vi "Main-loop-backup.vi"() -> ()   [LabVIEW 2016]
uses:
  Sched_state.ctl
  Plant_info.ctl
  <vilib>/Platform/TimedLoop/XDataNode/timing_clust.ctl
  <vilib>/Platform/TimedLoop/XDataNode/nitl_modes.ctl
  <vilib>/Platform/TimedLoop/XDataNode/wakeup.ctl
  <vilib>/Platform/TimedLoop/XDataNode/XDataNode.xnode
  <vilib>/Platform/TimedLoop/XDataNode/XDNodeRunTimeDep.lvlib
panel:
  out "error out":errorcluster
  out "loop time\n(only for diagnostics) - should be exactly 10, always":u32
  out "Plant 2 region":dbl(graph)
  out "Plant 1 region":dbl(graph)
  out "Plant 2":cluster{"Input":dbl, "Data":dbl, "Data":dbl}(graph)
  out "Plant 1":cluster{"Input":dbl, "Data":dbl, "Data":dbl}(graph)
  in  "error in (no error)":errorcluster
  in  "stop main":bool
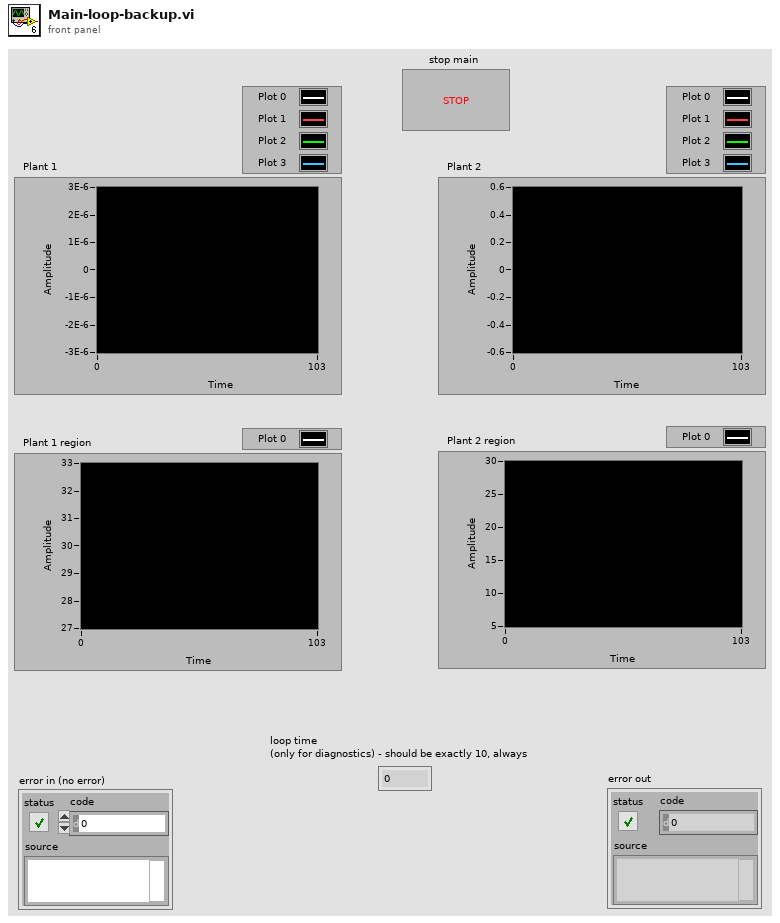
[diagram p1: front panel]
types:
  T1 = typedef "Sched_state.ctl" = cluster{"Plant 1":T2, "Plant 2":T2}
  T2 = typedef "Plant_info.ctl" = cluster{"Clk":dbl, "Region":dbl, "Input":dbl}
  T3 = typedef "Plant-data.ctl" = cluster{"Plant X1 ":dbl[], "Plant X2":dbl[], "Plant K*x_hat":dbl[], "Region":i32[]}
  T4 = typedef "XDNodeRunTimeDep.lvlib/timing_clust.ctl" = cluster{"Expected End [f-1]":u64, "Actual End [f-1]":u64, "Finished Late? [f-1]":bool, "Expected End [i-1]":u64, "Actual End [i-1]":u64, "Finished Late? [i-1]":bool, "Expected Start [i]":u64, "Actual Start [i]":u64, "Expected Start [f]":u64, "Actual Start [f]":u64, "Source Name":string, "Structure Name":string, "Period":i64, "Deadline":i64, "Offset":i64, "Start":i64, "Priority":i32, "Timeout":i32, "Mode":T5, "Wakeup Reason":T6, "Error":errorcluster, "Source Type":string, "Secondary Source Type":string, "Global End Time":u64, "Global Start Time":u64, "Frame Duration":u64, "Iteration Duration":u64, "Assigned CPU":i32, "I/O Scan Engine Mode":u32}
  T5 = typedef "XDNodeRunTimeDep.lvlib/nitl_modes.ctl" = enum32{"No Change", "Process missed periods, maintain original phase", "Discard missed periods, maintain original phase", "Process missed periods, ignore original phase", "Discard missed periods, ignore original phase"}
  T6 = typedef "XDNodeRunTimeDep.lvlib/wakeup.ctl" = enum32{"Normal", "Aborted", "Asynchronous wakeup", "Timing source error", "Timed loop error", "Timeout"}
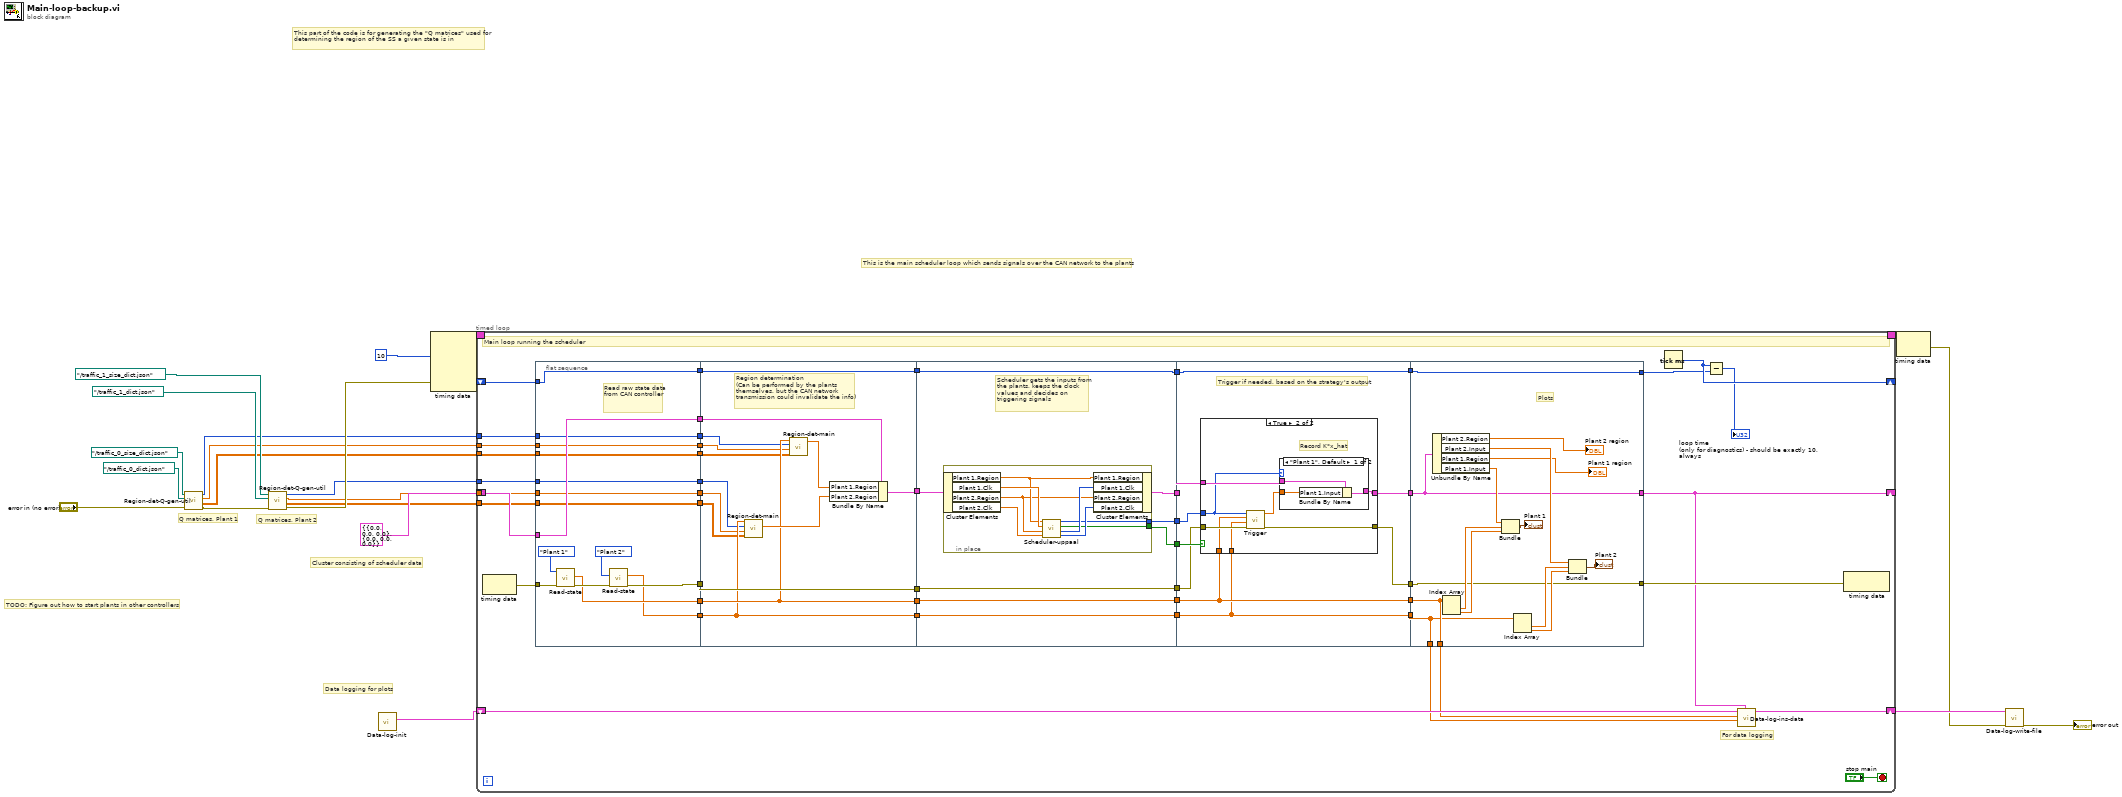
[diagram p0: block diagram]
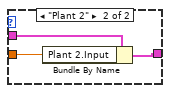
[diagram p3: hidden frame]
diagram:
  # "Data logging for plots"
  # "Q matrices, Plant 2"
  # "Q matrices, Plant 1"
  # "Cluster consisting of scheduler data"
  # "This part of the code is for generating the \"Q matrices\" used for determining the region of the SS a given state is in"
  # "TODO: Figure out how to start plants in other controllers"
  # "This is the main scheduler loop which sends signals over the CAN network to the plants"
  n1 = call "Region-det-Q-gen-util.vi"("error in"="error in (no error)", "Actual Q matrix JSON - rel path"=path "../traffic_0_dict.json", "Q matrix info JSON - rel path"=path "../traffic_0_size_dict.json") -> ("error out"=w13:errorcluster, "Q Matrices"=w6:dbl[][][][], "Index array"=w7:dbl[], "Regions"=w8:i32[])  [unwired: 5 in]
  n2 = call "Region-det-Q-gen-util.vi"("error in"=w13, "Actual Q matrix JSON - rel path"=path "../traffic_1_dict.json", "Q matrix info JSON - rel path"=path "../traffic_1_size_dict.json") -> ("error out"=w12:errorcluster, "Q Matrices"=w9:dbl[][][][], "Index array"=w5:dbl[], "Regions"=w10:i32[])  [unwired: 5 in]
  n3 = call "Data-log-init.vi"() -> ("Data cluster"=w4:cluster{"Plant 2":T3, "Plant 1":T3})  [unwired: 10 in, 1 out]
  n4 = node-c288(i64 10 ("Period"), w12) -> (w21:T4)  [unwired: 3 in]
  n5 = timed-loop {
    timing: w21 -> [_]
    timing-out: [_] -> w20
    shift-right: [w22] -> _
    shift-left: T1 {"Plant 1"={"Clk"=0.0, "Region"=0.0, "Input"=0.0}, "Plant 2"={"Clk"=0.0, "Region"=0.0, "Input"=0.0}} ("Scheduler State") -> [w65]
    tunnel: w10 -> [w47]
    tunnel: w5 -> [w44]
    tunnel: w9 -> [w42]
    tunnel: w8 -> [w40]
    tunnel: w7 -> [w39]
    tunnel: w6 -> [w36]
    shift-right: [w34] -> _
    shift-left: _ -> [w32]
    shift-right: [w25] -> w3
    shift-left: w4 -> [w26]
    stop <- "stop main" stop-if-true
    # "For data logging"
    # "Main loop running the scheduler"
    n6 = node-c288() -> (w68:errorcluster)  [unwired: 1 in]
    n7 = flat-sequence {
      tunnel: w68 -> [w81]
      tunnel: w65 -> [w78]
      tunnel: [w78] -> w56
      tunnel: [w79] -> w52
      tunnel: [w77] -> w49
      tunnel: [w76] -> w48
      tunnel: w47 -> [w75]
      tunnel: [w75] -> w46
      tunnel: [w74] -> w45
      tunnel: w44 -> [w74]
      tunnel: [w73] -> w43
      tunnel: w42 -> [w73]
      tunnel: [w72] -> w41
      tunnel: w40 -> [w72]
      tunnel: w39 -> [w71]
      tunnel: [w71] -> w38
      tunnel: w36 -> [w70]
      tunnel: [w70] -> w37
      tunnel: w32 -> [w69]
      tunnel: [w69] -> w31
      tunnel: [w92] -> w62
      tunnel: [w91] -> w59
      tunnel: w56 -> [w97]
      tunnel: [w94] -> w55
      tunnel: [w93] -> w53
      tunnel: w52 -> [w93]
      tunnel: w49 -> [w92]
      tunnel: w48 -> [w91]
      tunnel: w46 -> [w90]
      tunnel: w45 -> [w89]
      tunnel: w43 -> [w88]
      tunnel: w41 -> [w87]
      tunnel: w38 -> [w85]
      tunnel: w37 -> [w86]
      tunnel: w31 -> [w84]
      tunnel: [w84] -> w30
      tunnel: [w105] -> w64
      tunnel: [w99] -> w63
      tunnel: w62 -> [w104]
      tunnel: [w104] -> w61
      tunnel: [w103] -> w60
      tunnel: w59 -> [w103]
      tunnel: [w102] -> w57
      tunnel: w55 -> [w101]
      tunnel: [w100] -> w54
      tunnel: w53 -> [w100]
      tunnel: w30 -> [w98]
      tunnel: [w98] -> w28
      tunnel: [w119] -> w67
      tunnel: w64 -> [w115]
      tunnel: w63 -> [w120]
      tunnel: w61 -> [w117]
      tunnel: w60 -> [w116]
      tunnel: [w121] -> w58
      tunnel: w57 -> [w122]
      tunnel: w54 -> [w118]
      tunnel: [w116] -> w51
      tunnel: [w117] -> w50
      tunnel: [w114] -> w29
      tunnel: w28 -> [w114]
      tunnel: w67 -> [w143]
      tunnel: [w142] -> w22
      tunnel: w58 -> [w142]
      tunnel: w51 -> [w139]
      tunnel: w50 -> [w140]
      tunnel: [w143] -> w35
      tunnel: [w141] -> w33
      tunnel: w29 -> [w141]
      tunnel: [w140] -> w24
      tunnel: [w139] -> w23
      frame #0 {
        # "Read raw state data from CAN controller"
        n8 = call "Read-state.vi"("error in (no error)"=w81, "Plant"=enum16{"Plant 1", "Plant 2"}."Plant 1") -> ("error out"=w80:errorcluster, "state"=w77:dbl[])  [unwired: 8 in]
        n9 = call "Read-state.vi"("error in (no error)"=w80, "Plant"=enum16{"Plant 1", "Plant 2"}."Plant 2") -> ("error out"=w79:errorcluster, "state"=w76:dbl[])  [unwired: 8 in]
      }
      frame #1 {
        # "Region determination \n(Can be performed by the plants\nthemselves, but the CAN network \ntransmission could invalidate the info)"
        n10 = call "Region-det-main.vi"("Q Matrices"=w88, "Index Array"=w89, "Regions"=w90, "State"=w91) -> ("Region"=w95:dbl)  [unwired: 7 in]
        n11 = call "Region-det-main.vi"("Q Matrices"=w86, "Index Array"=w85, "Regions"=w87, "State"=w92) -> ("Region"=w96:dbl)  [unwired: 7 in]
        n12 = Bundle By Name(cluster=w97, "Plant 1.Region"=w96, "Plant 2.Region"=w95) -> (w94:T1)
      }
      frame #2 {
        # "Scheduler gets the inputs from the plants, keeps the clock values and decides on triggering signals"
        n13 = in-place {
          in-place-border: [w111] -> w105
          in-place-border: [w110] -> w99
          n14 = in-place-cluster #1(w101) -> ("Plant 1.Region"=w107:dbl, "Plant 1.Clk"=w109:dbl, "Plant 2.Region"=w106:dbl, "Plant 2.Clk"=w108:dbl)
          n15 = call "Scheduler-uppaal.vi"("Clock, plant 2"=w108, "Region, plant 2"=w106, "Clock, plant 1"=w109, "Region, plant 1"=w107) -> ("Clock 2"=w112:i32, "Clock 1"=w113:i32, "Trigger?"=w110:bool, "Plant to trigg"=w111:enum16{"Plant 1", "Plant 2"})  [unwired: 4 in]
          n16 = in-place-cluster #1("Plant 1.Region"=w107, "Plant 1.Clk"=w113, "Plant 2.Region"=w106, "Plant 2.Clk"=w112) -> (w102:T1)
        }
      }
      frame #3 {
        # "Trigger if needed, based on the strategy's output"
        n17 = case shown="True" w120 {
          tunnel: w122 -> [w124 w129]
          tunnel: [w124 w130] -> w121
          tunnel: w117 -> [_ w126]
          tunnel: w118 -> [w123 w132]
          tunnel: [w123 w131] -> w119
          tunnel: w115 -> [_ w128]
          tunnel: w116 -> [_ w125]
          frame False {
          }
          frame True {
            # "Record K*x_hat"
            n18 = call "Trigger.vi"("error in (no error)"=w132, "State, Plant 2"=w125, "State, Plant 1"=w126, "Plant to trigg"=w128) -> ("error out"=w131:errorcluster, "Kx"=w127:dbl)  [unwired: 6 in]
            n19 = case shown="\"Plant 1\", Default" w128 {
              tunnel: [w133 w138] -> w130
              tunnel: w129 -> [w135 w137]
              tunnel: w127 -> [w134 w136]
              frame "Plant 1", Default {
                n20 = Bundle By Name(cluster=w135, "Plant 1.Input"=w134) -> (w133:T1)
              }
              frame "Plant 2" {
                n21 = Bundle By Name(cluster=w137, "Plant 2.Input"=w136) -> (w138:T1)
              }
            }
          }
        }
      }
      frame #4 {
        # "Plots"
        n22 = Unbundle By Name(w142) -> ("Plant 2.Region"=→"Plant 2 region":dbl, "Plant 2.Input"=w149:dbl, "Plant 1.Region"=→"Plant 1 region":dbl, "Plant 1.Input"=w148:dbl)
        n23 = Index Array(array=w140) -> (element #1=w153:dbl, element #2=w152:dbl)  [unwired: 2 in]
        n24 = Bundle("Input"=w148, "Data"=w153, "Data"=w152) -> (→"Plant 1":cluster{"Input":dbl, "Data":dbl, "Data":dbl})  [unwired: 1 in]
        n25 = Index Array(array=w139) -> (element #1=w151:dbl, element #2=w150:dbl)  [unwired: 2 in]
        n26 = Bundle("Input"=w149, "Data"=w151, "Data"=w150) -> (→"Plant 2":cluster{"Input":dbl, "Data":dbl, "Data":dbl})  [unwired: 1 in]
      }
    }
    n27 = Tick Count (ms)() -> (millisecond timer value=w34:u32)
    n28 = Subtract(x=w34, y=w33) -> (x-y=→"loop time\n(only for diagnostics) - should be exactly 10, always":u32)
    n29 = call "Data-log-ins-data.vi"("Scheduler State"=w22, "Plant 2 State"=w23, "Plant 1 State"=w24, "Data cluster in"=w26) -> ("Data cluster out"=w25:cluster{"Plant 2":T3, "Plant 1":T3})  [unwired: 7 in]
    n30 = node-c288(w35) -> ()  [unwired: 1 out]
  }
  n31 = node-c288(w20) -> (w1:errorcluster)
  n32 = call "Data-log-write-file.vi"("error in (no error)"=w1, "Data cluster in"=w3) -> ("error out"=→"error out":errorcluster)  [unwired: 9 in]
